vi "JKI Arguments to Array.vi"(0 "Arguments":string, 1 "Delimiter (,)":string=",") -> (4 "Argument":string[](array[string]))   [LabVIEW 2017]
uses:
  <vilib>/Utility/error.llb/whitespace.ctl
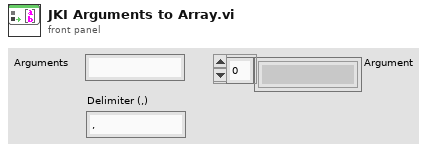
[diagram p1: front panel]
types:
  T1 = typedef "whitespace.ctl" = u16
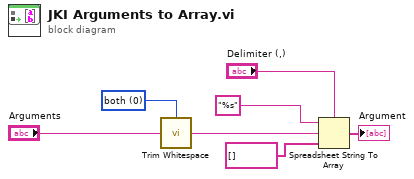
[diagram p0: block diagram]
diagram:
  w4 = T1 0 items=["both", "start of string", "end of string"] ("location (both)")
  n1 = call <vilib>:"Trim Whitespace.vi"("string"="Arguments", "location (both)"=w4) -> ("trimmed string"=w2:string)
  n2 = Spreadsheet String To Array ("电子表格字符串至数组转换")(delimiter (Tab)="Delimiter (,)", format string="%s" ("格式字符串"), spreadsheet string=w2, array type (2D Dbl)=string[] []) -> (array=→"Argument":string[])
